vi "Escape_Json.vi"(10 "String":string="hola\nvamos a probar\nsi esto tiene efecto o no  \\ \ny con comillas y todo \"") -> (3 "Json_string":string)   [LabVIEW 2014]
panel:
  # "Escape offending characters \\ \\n \\t\""
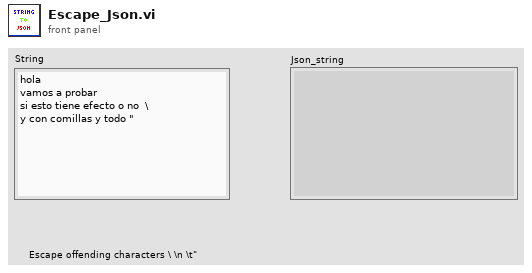
[diagram p1: front panel]
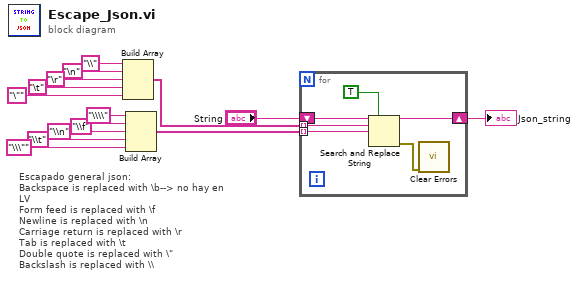
[diagram p0: block diagram]
diagram:
  # "Escapado general json:\nBackspace is replaced with \\b--> no hay en LV\nForm feed is replaced with \\f\nNewline is replaced with \\n\nCarriage return is replaced with \\r\nTab is replaced with \\t \nDouble quote is replaced with \\\"\nBackslash is replaced with \\\\"
  n1 = Build Array("\\" ("replace string (\"\")"), "\n", "\r", "\t", "\"") -> (w4:string[])
  n2 = Build Array("\\\\" ("replace string (\"\")"), "\\f" ("replace string (\"\")"), "\\n" ("replace string (\"\")"), "\\t" ("replace string (\"\")"), "\\\"") -> (w3:string[])
  n3 = for {
    tunnel: w4 -> [w19] mode=indexing
    tunnel: w3 -> [w18] mode=indexing
    shift-right: [w17] -> w1
    shift-left: "String" -> [w16]
    n4 = Search and Replace String(replace all?=TRUE ("replace all? (F)"), input string=w16, search string=w19, replace string=w18) -> (result string=w17:string, error out=w15:errorcluster)  [unwired: 4 in, 2 out]
    n5 = call <vilib>:"Clear Errors.vi"("error in (no error)"=w15) -> ()  [unwired: 5 in, 2 out]
  }
  "Json_string" <- w1
